vi "Temperature Warnings.vi"(8 "error in (no error)":errorcluster, 9 "Min Temperature":dbl, 10 "Max Temperature":dbl, 11 "Current Temperature":dbl) -> (0 "error out":errorcluster, 2 "Warning Text":string="No Warning", 3 "Warning?":bool)   [LabVIEW 2015]
doc: "This VI is used to determine the string to output to the weather station based on the current temperature and limit settings.\n\nInputs: Current Temperature (DBL), Minimum Temperature (DBL), and Maximum Temperature (DBL).\nOutputs: Warning Text (string) and Warning? (Boolean)."
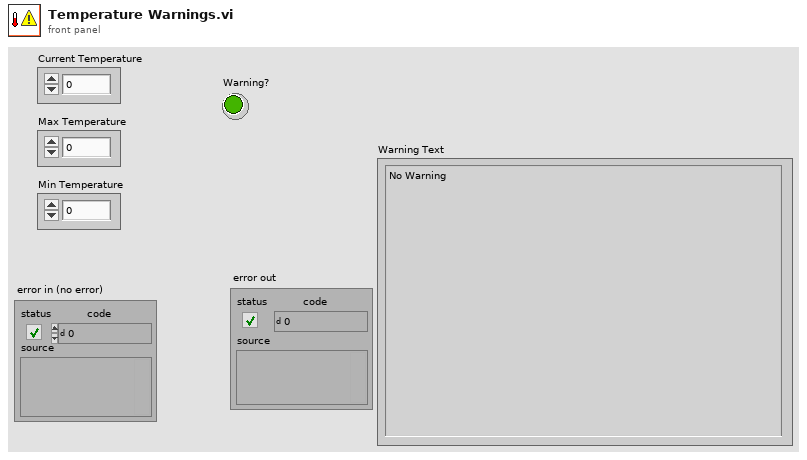
[diagram p1: front panel]
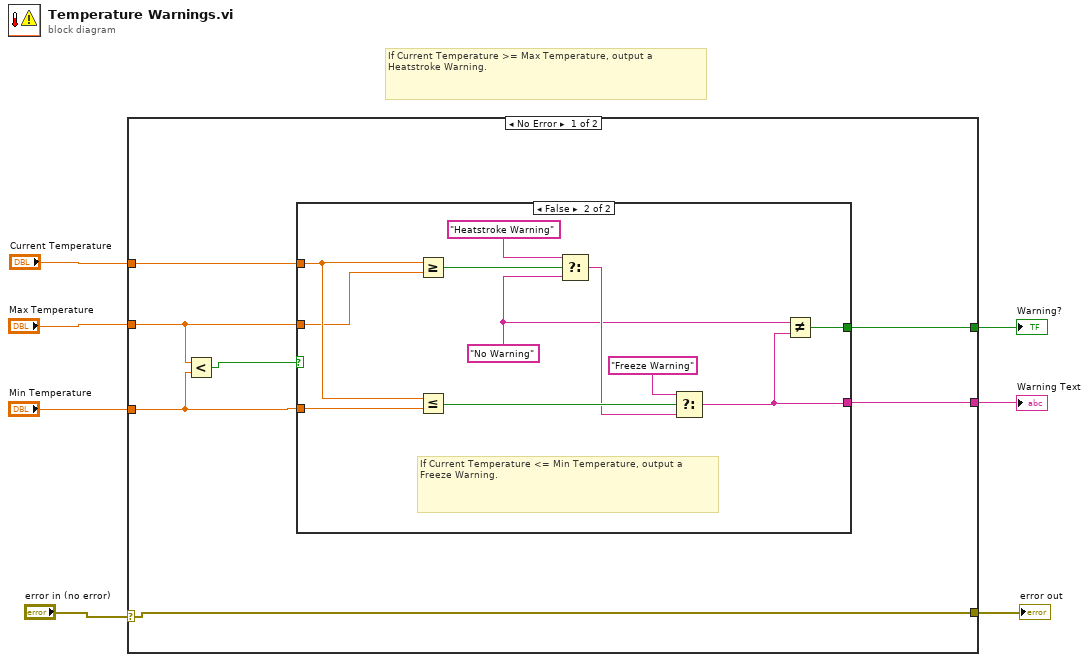
[diagram p0: block diagram]
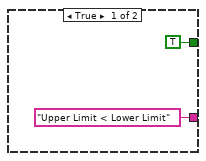
[diagram p2: hidden frame]
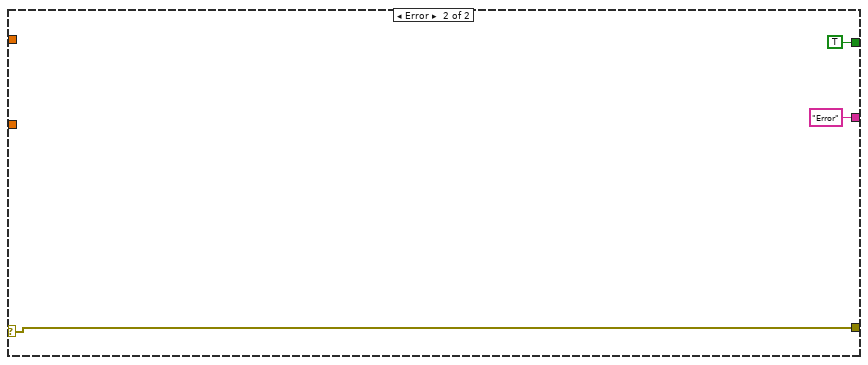
[diagram p3: hidden frame]
diagram:
  # "If Current Temperature >= Max Temperature, output a Heatstroke Warning."
  n1 = case shown="No Error" "error in (no error)" {
    selector: "error in (no error)" -> [w11 w28]
    tunnel: "Current Temperature" -> [w14 _]
    tunnel: "Min Temperature" -> [w9 _]
    tunnel: "Max Temperature" -> [w10 _]
    tunnel: [w13 TRUE] -> w4
    tunnel: [w12 "Error" ("f")] -> w3
    tunnel: [w11 w28] -> w1
    frame No Error {
      n2 = Less?(x=w10, y=w9) -> (x < y?=w8:bool)
      n3 = case shown="False" w8 {
        tunnel: w14 -> [_ w27]
        tunnel: w9 -> [_ w26]
        tunnel: w10 -> [_ w25]
        tunnel: [TRUE w24] -> w13
        tunnel: ["Upper Limit < Lower Limit" ("f") w23] -> w12
        frame True {
        }
        frame False {
          w17 = "No Warning" ("f")
          # "If Current Temperature <= Min Temperature, output a Freeze Warning."
          n4 = Greater Or Equal?(x=w27, y=w25) -> (x >= y?=w22:bool)
          n5 = Less Or Equal?(x=w27, y=w26) -> (x <= y?=w19:bool)
          n6 = Select(t="Heatstroke Warning", s=w22, f=w17) -> (s? t:f=w18:string)
          n7 = Select(t="Freeze Warning", s=w19, f=w18) -> (s? t:f=w23:string)
          n8 = Not Equal?(x=w17, y=w23) -> (x != y?=w24:bool)
        }
      }
    }
    frame Error {
    }
  }
  "Warning?" <- w4
  "Warning Text" <- w3
  "error out" <- w1
